vi "ControlPlans.vi"(8 "error in (no error)":errorcluster, 11 "ByteQXAPIBase in":refnum<class "ByteQXAPIBase.lvclass">) -> (0 "error out":errorcluster, 2 "Values":T1[](array[typedef]), 3 "ByteQXAPIBase out":refnum<class "ByteQXAPIBase.lvclass">)   [LabVIEW 2019, in "ByteQXWebAPI.lvlib" / "ByteQXAPIBase.lvclass"]
uses:
  ByteQXAPIBase.lvclass
  ControlPlan.ctl
  Private/module.ctl
  ByteQXAPIBase.lvclass/ByteQXAPIBase.ctl
  <vilib>/Bytelabs/ByteREST/ByteRESTClass/ByteRESTBase/RESTBase.lvclass
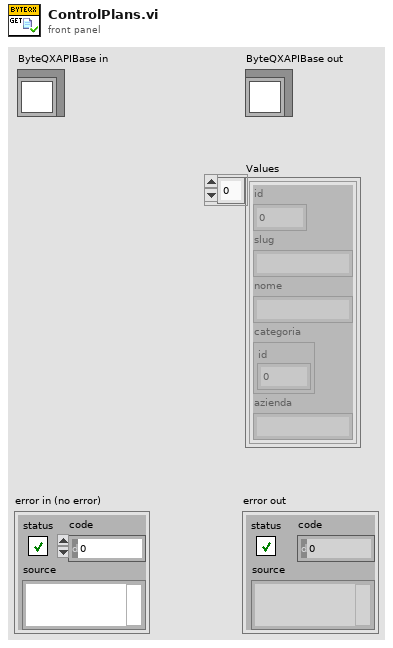
[diagram p1: front panel]
types:
  T1 = typedef "ByteQXWebAPI.lvlib/ByteQXAPIBase.lvclass/ControlPlan.ctl" = cluster{"id":i32, "slug":string, "nome":string, "categoria":cluster{"id":i32}, "azienda":string}
  T2 = typedef "ByteQXWebAPI.lvlib/ByteQXAPIBase.lvclass/module.ctl" = enum16{"gs", "tms"}
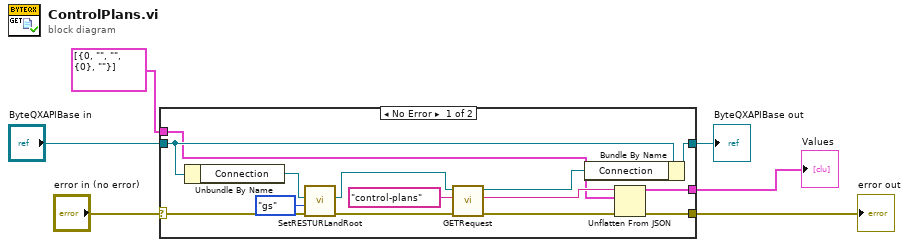
[diagram p0: block diagram]
diagram:
  n1 = case shown="No Error" "error in (no error)" {
    selector: "error in (no error)" -> [w11 w23]
    tunnel: [w12 w23] -> w3
    tunnel: T1[] [{"id"=0, "slug"="", "nome"="", "categoria"={"id"=0}, "azienda"=""}] -> [w14 w22]
    tunnel: [w13 w22] -> w1
    tunnel: [w18 w21] -> w4
    tunnel: "ByteQXAPIBase in" -> [w20 w21]
    frame No Error {
      n2 = Unbundle By Name(w20) -> ("Connection"=w9:refnum<class "RESTBase.lvclass">)
      n3 = call "SetRESTURLandRoot.vi"("error in (no error)"=w11, "module"=module."gs", "ByteREST in"=w9) -> ("error out"=w10:errorcluster, "ByteREST out"=w8:refnum<class "RESTBase.lvclass">)  [unwired: 7 in]
      n4 = call-dynamic "GETRequest.vi"("error in (no error)"=w10, "Request"="control-plans", "ByteRESTBase in"=w8) -> ("error out"=w19:errorcluster, "Body"=w15:string, "ByteRESTBase out"=w17:refnum<class "RESTBase.lvclass">)  [unwired: 5 in, 1 out]
      n5 = Bundle By Name(cluster=w20, "Connection"=w17) -> (w18:refnum<class "ByteQXAPIBase.lvclass">)
      n6 = Unflatten From JSON(JSON string=w15, type and defaults=w14, error in (no error)=w19) -> (value=w13:T1[], error out=w12:errorcluster)  [unwired: 4 in]
    }
    frame Error {
    }
  }
  "error out" <- w3
  "ByteQXAPIBase out" <- w4
  "Values" <- w1
